vi "SaveTankData.vi"(0 "Log Pressure":bool, 1 "4He Pressure (Torr)":string, 2 "3He Pressure (Torr)":string) -> ()   [LabVIEW 2018]
panel:
  out "error out":errorcluster
  in  "Data folder":path=path "C:/Data"
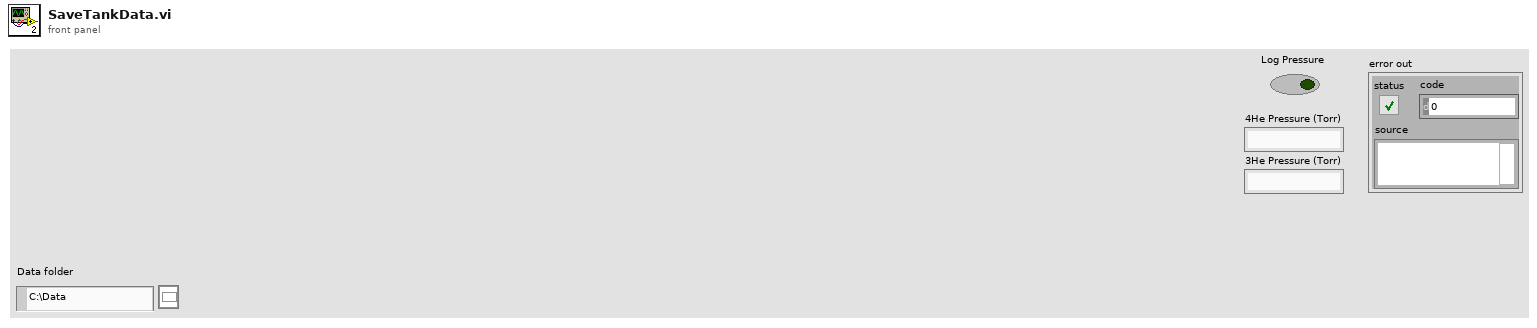
[diagram p1: front panel]
types:
  T1 = enum16{"open", "replace", "create", "open or create", "replace or create", "replace or create with confirmation"}
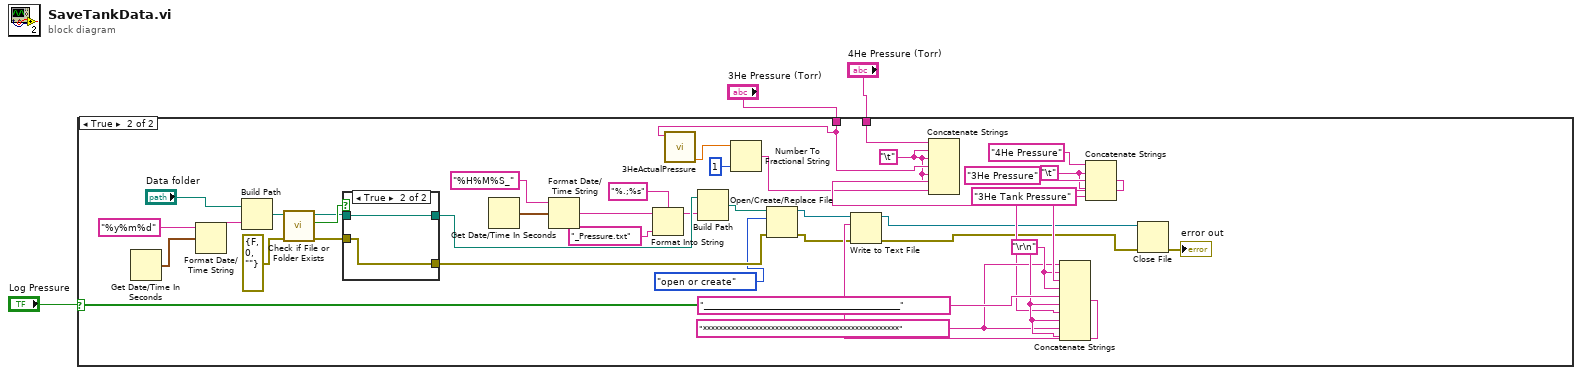
[diagram p0: block diagram]
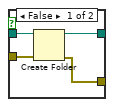
[diagram p3: hidden frame]
diagram:
  n1 = case shown="True" "Log Pressure" {
    tunnel: "4He Pressure (Torr)" -> [_ w11]
    tunnel: "3He Pressure (Torr)" -> [_ w9]
    frame False {
    }
    frame True {
      w7 = "\t"
      w5 = "\t"
      w37 = "*************************************************" ("string")
      w38 = "\r\n"
      n2 = Get Date/Time In Seconds() -> (seconds since 1Jan1904=w24:timestamp)
      n3 = Format Date/Time String(time format string (%c)="%y%m%d", seconds (now)=w24) -> (date/time string=w25:string)  [unwired: 1 in]
      n4 = Build Path(base path="Data folder", name or relative path=w25) -> (appended path=w26:path)
      n5 = call "Check if File or Folder Exists.vi"("error in (no error)"=errorcluster {"status"=FALSE, "code"=0, "source"=""}, "path"=w26) -> ("error out"=w33:errorcluster, "file or folder exists?"=w28:bool, "dup path"=w27:path)  [unwired: 7 in]
      n6 = case shown="True" w28 {
        tunnel: w27 -> [w47 w49]
        tunnel: [w46 w49] -> w32
        tunnel: w33 -> [w45 w48]
        tunnel: [w44 w48] -> w35
        frame False {
          n7 = Create Folder(path (use dialog)=w47, error in=w45) -> (created path=w46:path, error out=w44:errorcluster)  [unwired: 1 in, 1 out]
        }
        frame True {
        }
      }
      n8 = Get Date/Time In Seconds() -> (seconds since 1Jan1904=w29:timestamp)
      n9 = Format Date/Time String(time format string (%c)="%H%M%S_", seconds (now)=w29) -> (date/time string=w31:string)  [unwired: 1 in]
      n10 = Format Into String(format string="%.;%s", initial string=w31, "_Pressure.txt" ("input 2")) -> (resulting string=w30:string)  [unwired: 1 in, 1 out]
      n11 = call "3HeActualPressure.vi"("3He Pressure (Torr)"=w9) -> ("Actual 3He\nTank Pressure"=w10:dbl)  [unwired: 10 in]
      n12 = Build Path(base path=w32, name or relative path=w30) -> (appended path=w34:path)
      n13 = Number To Fractional String(number=w10, precision (6)=i16 1) -> (F-format string=w6:string)  [unwired: 2 in]
      n14 = Open/Create/Replace File(file path (use dialog)=w34, error in=w35, operation (0:open)=T1."open or create") -> (refnum out=w15:refnum<file>, error out=w16:errorcluster)  [unwired: 3 in, 1 out]
      n15 = Concatenate Strings(w11, w7, w7, w9, w7, w7, w6) -> (w36:string)
      n16 = Concatenate Strings("4He Pressure" ("string"), w5, "3He Pressure" ("string"), w5, "3He Tank Pressure" ("string")) -> (w39:string)
      n17 = Concatenate Strings(w37, w38, w39, w38, "_________________________________________________" ("string"), w38, w36, w38, w37, w38) -> (w43:string)
      n18 = Write to Text File(file (use dialog)=w15, text=w43, error in=w16) -> (refnum out=w13:refnum<file>, error out=w12:errorcluster)  [unwired: 1 in, 1 out]
      n19 = Close File(refnum=w13, error in=w12) -> (error out=→"error out":errorcluster)  [unwired: 1 out]
    }
  }
